vi "ECOG-Update Display.vi"(0 "display in":T1 {"IIR Filter"."Forward Coefficients" format="%.4f"; "IIR Filter"."Reverse Coefficients" format="%.4f"}, 7 "new data":dbl[](array[numeric])) -> (4 "display out":T1 {"IIR Filter"."Forward Coefficients" format="%.4f"; "IIR Filter"."Reverse Coefficients" format="%.4f"})   [LabVIEW 2020]
uses:
  Typedefs/ECOG-Display.ctl
  5e1dc45d-3397-4ae4-9168-812a6a074c8d.vi
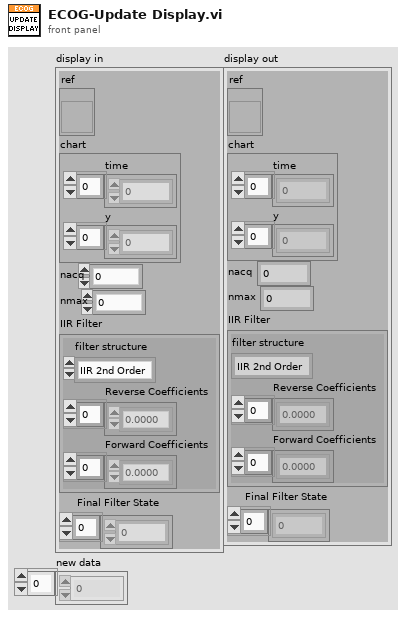
[diagram p1: front panel]
types:
  T1 = typedef "ECOG-Display.ctl" = cluster{"ref":refnum<vi>, "chart":cluster{"time":dbl[], "y":dbl[]}, "nacq":i32, "nmax":i32, "IIR Filter":cluster{"filter structure":enum32{"IIR 2nd Order", "IIR 4th Order"}, "Reverse Coefficients":dbl[], "Forward Coefficients":dbl[]}, "Final Filter State":dbl[]}
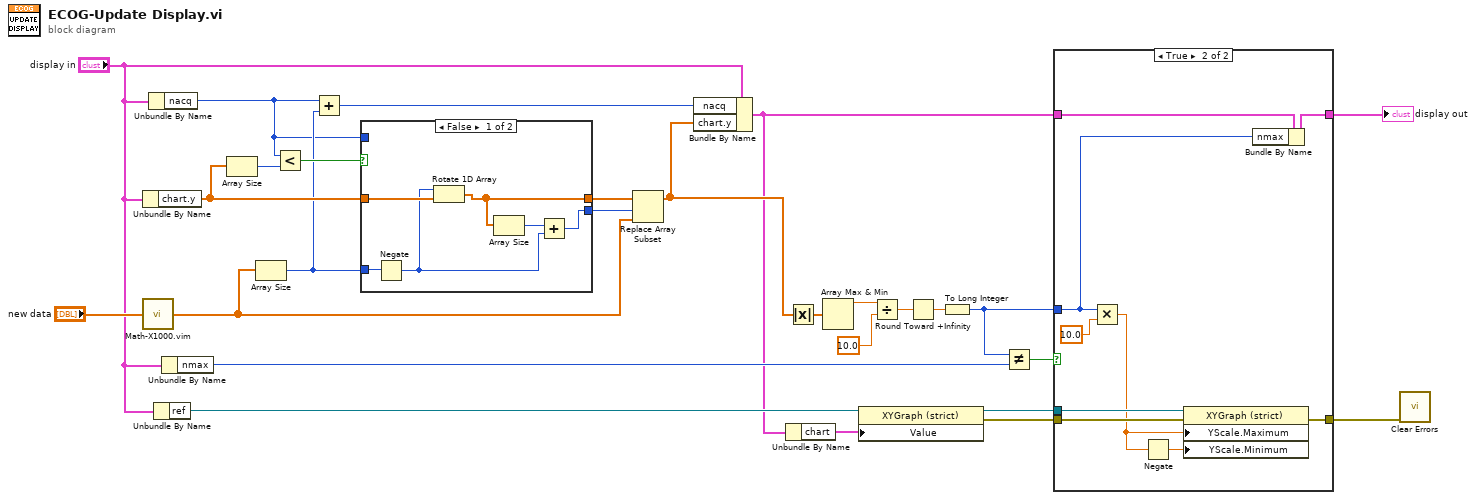
[diagram p0: block diagram]
diagram:
  n1 = Unbundle By Name("display in") -> ("chart.y"=w26:dbl[])
  n2 = call "Math-X1000.vim"("X"="new data") -> ("1000X"=w1:dbl[])
  n3 = Unbundle By Name("display in") -> ("nacq"=w21:i32)
  n4 = Unbundle By Name("display in") -> ("ref"=w19:refnum<vi>)
  n5 = Unbundle By Name("display in") -> ("nmax"=w10:i32)
  n6 = Array Size(array=w26) -> (size(s)=w27:i32)
  n7 = Array Size(array=w1) -> (size(s)=w24:i32)
  n8 = Less?(x=w21, y=w27) -> (x < y?=w25:bool)
  n9 = Add(x=w21, y=w24) -> (x+y=w23:i32)
  n10 = case shown="False" w25 {
    tunnel: w26 -> [w32 w35]
    tunnel: [w31 w35] -> w22
    tunnel: w24 -> [w33 _]
    tunnel: w21 -> [_ w34]
    tunnel: [w28 w34] -> w20
    frame False {
      n11 = Negate(x=w33) -> (-x=w29:i32)
      n12 = Rotate 1D Array(1:w32, 2:w29) -> (0:w31:dbl[])
      n13 = Array Size(array=w31) -> (size(s)=w30:i32)
      n14 = Add(x=w30, y=w29) -> (x+y=w28:i32)
    }
    frame True {
    }
  }
  n15 = Replace Array Subset(array=w22, new element=w1, index=w20) -> (w13:dbl[])
  n16 = Bundle By Name(cluster="display in", "nacq"=w23, "chart.y"=w13) -> (w4:T1)
  n17 = Unbundle By Name(w4) -> ("chart"=w18:cluster{"time":dbl[], "y":dbl[]})
  n18 = Absolute Value(x=w13) -> (abs(x)=w12:dbl[])
  n19 = Array Max & Min(array=w12) -> (max value=w2:dbl)  [unwired: 3 out]
  n20 = property class="XYGraph (strict)"(reference=w19, "Value"=w18) -> (reference out=w9:refnum<vi>, error out=w7:errorcluster)  [unwired: 1 in]
  n21 = Divide(x=w2, y=10.0) -> (x/y=w16:dbl)
  n22 = Round Toward +Infinity(x=w16) -> (ceil(x): smallest int >= x=w17:dbl)
  n23 = To Long Integer(number=w17) -> (32bit integer=w6:i32)
  n24 = Not Equal?(x=w6, y=w10) -> (x != y?=w8:bool)
  n25 = case shown="True" w8 {
    tunnel: w9 -> [_ w46]
    tunnel: w7 -> [w37 w45]
    tunnel: w6 -> [_ w38]
    tunnel: [w37 w41] -> w5
    tunnel: w4 -> [w36 w40]
    tunnel: [w36 w39] -> w3
    frame False {
    }
    frame True {
      n26 = Multiply(x=w38, y=10.0) -> (x*y=w42:dbl)
      n27 = Negate(x=w42) -> (-x=w43:dbl)
      n28 = property class="XYGraph (strict)"(reference=w46, error in=w45, "YScale.Maximum"=w42, "YScale.Minimum"=w43) -> (error out=w41:errorcluster)  [unwired: 1 out]
      n29 = Bundle By Name(cluster=w40, "nmax"=w38) -> (w39:T1)
    }
  }
  "display out" <- w3
  n30 = call <vilib>:"Clear Errors.vi"("error in (no error)"=w5) -> ()  [unwired: 5 in, 2 out]
